vi "Memory.Pointer.Swap.vi"   [LabVIEW 2016, in "Memory.lvlib" / "Memory.Pointer.lvclass"]
doc: "Swaps the address of the two provided <b>pointers</b>. This cannot be used with external pointers created via the Encapsulate method.\n\n<b>Safe:</b>\nThe size of both pointers must be the same, or a runtime error is thrown.\n\n<b>Unsafe:</b>\nNo size check is performed."
uses:
  Memory.Pointer.lvclass
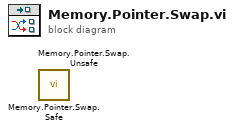
[diagram p0: block diagram]
diagram:
  n1 = call "Memory.Pointer.Swap.Safe.vi"() -> ()  [unwired: 9 in, 3 out]
  n2 = call "Memory.Pointer.Swap.Unsafe.vi"() -> ()  [unwired: 9 in, 3 out]
